vi "Counter (SubVI).vi"(9 "Input Valid":bool=TRUE, 10 "Counter End  Value":u32, 11 "Reset":bool) -> (2 "Counter Value":u32, 3 "End Reached":bool)   [LabVIEW 2015]
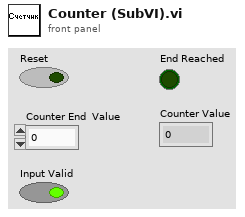
[diagram p1: front panel]
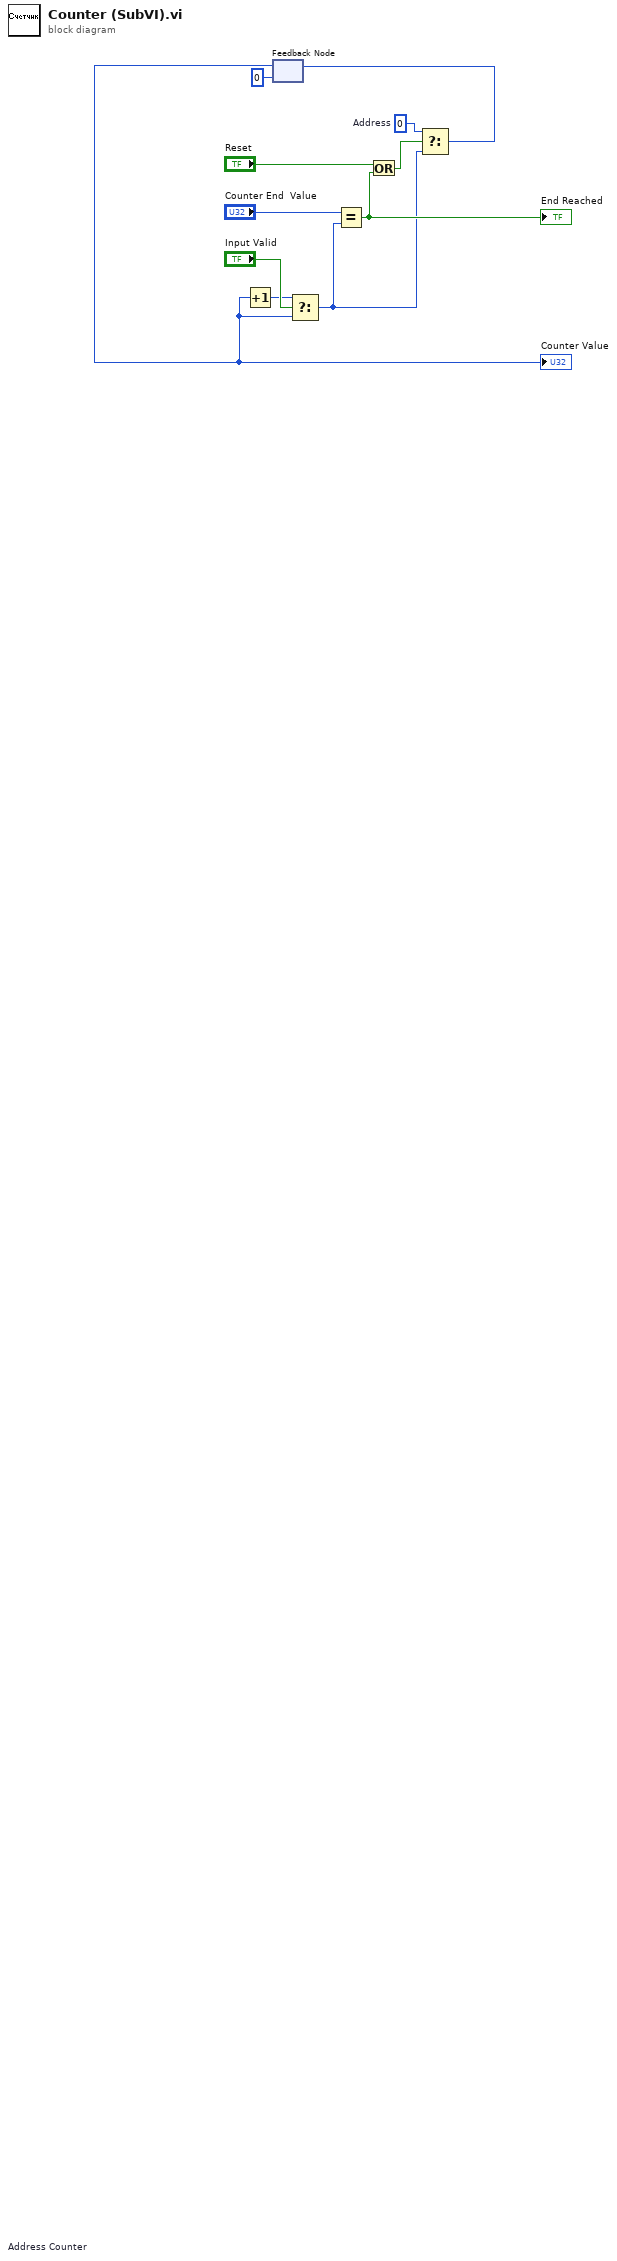
[diagram p0: block diagram]
diagram:
  w1 = u32 0  # Address
  n1 = feedback #1 "Address Counter"(u32 0 ("Address")) -> (w8:u32)
  "Counter Value" <- w8
  n2 = Increment(x=w8) -> (x+1=w4:u32)
  n3 = Select(t=w4, s="Input Valid", f=w8) -> (s? t:f=w5:u32)
  n4 = Equal?(x="Counter End  Value", y=w5) -> (x = y?=w10:bool)
  "End Reached" <- w10
  n5 = Or(x="Reset", y=w10) -> (x .or. y?=w9:bool)
  n6 = Select(t=w1, s=w9, f=w5) -> (s? t:f=w2:u32)
  n7 = feedback-in #1(w2) -> ()
